vi "OutputSwerveAzimuth.vi"() -> ()   [LabVIEW 2020]
doc: "This VI runs feedback and feedforward controllers, manages safety interlocks, and sends commands to the swerve azimuth motors."
uses:
  <vilib>/Rock Robotics/WPI/ThirdParty/Phoenix-LabVIEW/Motor Controller/Controls/CTRE_Phoenix_MotorControl_ControlMode.ctl
  <vilib>/Rock Robotics/WPI/ThirdParty/Phoenix-LabVIEW/Motor Controller/Controls/CTRE_Phoenix_MotorControl_NeutralMode.ctl
  6e813111-160f-47d9-be7e-04f12fb0a952.vi
  refnumbers.vi
  GRNF_CTREMotor.vi
  sensordata.vi
  driverdata.vi
  robotoutputs.vi
  robotconstants.vi
  TAI_Motor.vi
  <vilib>/Rock Robotics/WPI/ThirdParty/Phoenix-LabVIEW/Motor Controller/Get/CTRE_Phoenix_MotorController_GetSelectedSensorData.vi
panel:
  out "Azimuth Error (deg)":dbl
  out "Azimuth Velocity":cluster{dbl}(graph)
  out "Azimuth Position":cluster{dbl, "Interlock Output":dbl}(graph)
  in  "PID Parameters":T1={"Kp"=0.3, "Ki"=0.0, "Kd"=0.0, "Kf (don't use)"=0.0, "I-Zone"=10.0} {"Kd" min=0.0; "Ki" min=0.0; "Kp" min=0.0}
  in  "S-Curve Strength":i32=4
  in  "Acceleration (deg/s^2)":dbl=10000.0
  in  "Cruise Velocity (deg/s)":dbl=1000.0
  in  "Manual Azimuth Goal (deg) [-180,180]":dbl
  in  "Manually Override Azimuth Goal":bool
  in  "Best Angle Hysteresis (deg)":dbl=20.0 format="%#_13g"
  in  "Plotting":T2(ring)
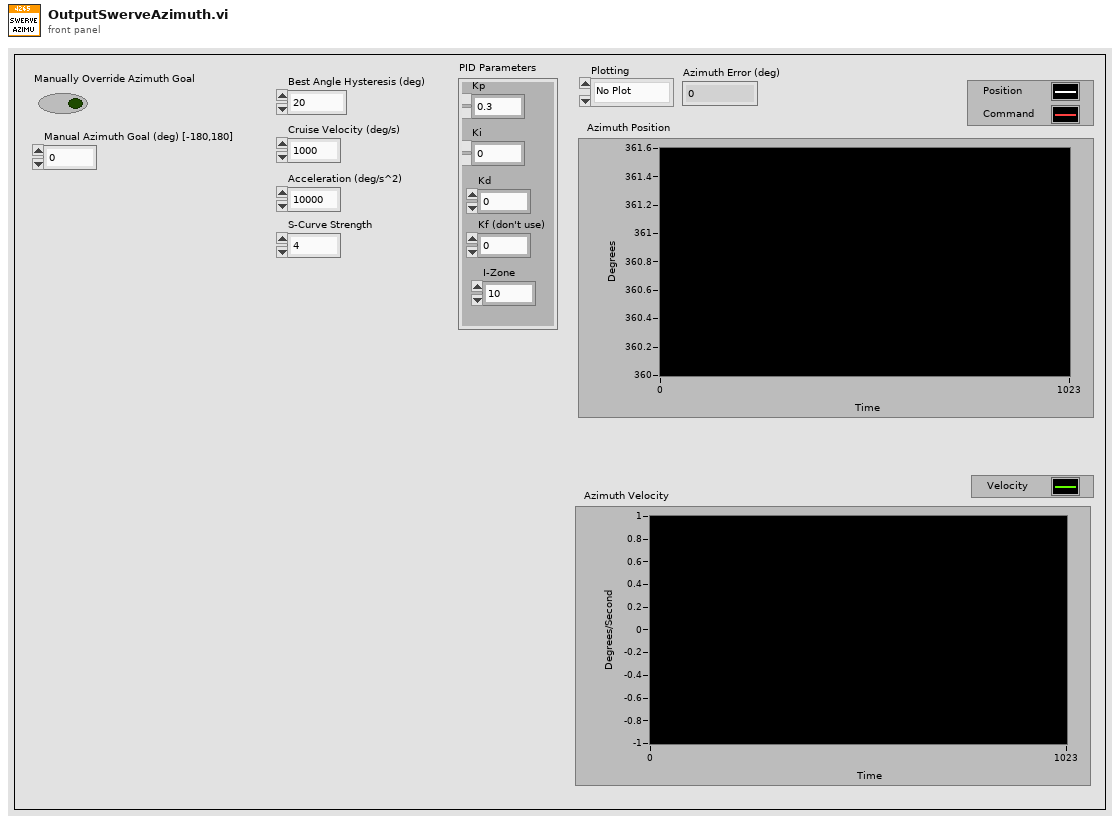
[diagram p1: front panel]
types:
  T1 = cluster{"Kp":dbl, "Ki":dbl, "Kd":dbl, "Kf (don't use)":dbl, "I-Zone":dbl}
  T2 = enum16{"No Plot", "Module 0", "Module 1", "Module 2", "Module 3"}
  T3 = cluster{"Cruise Velocity (deg/s)":i32, "Acceleration (deg/s^2)":i32, "S-Curve Strength":i32}
  T4 = cluster{"Cruise Velocity (deg/s)":bool, "Acceleration (deg/s^2)":bool, "S-Curve Strength":bool}
  T5 = cluster{"Kp":bool, "Ki":bool, "Kd":bool, "Kf (don't use)":bool, "I-Zone":bool}
  T6 = typedef "WPI_MotorControlDeviceRef.ctl" = cluster{"DeviceStatus":errorcluster, "Type":T7, "PWM":cluster{"PWM Channel":T8, "DeadBand":T9}, "CAN":cluster{"Device Number":u8, "SetOutput VI Ref":variant, "GetOutput VI Ref":variant, "Enable VI Ref":variant, "Disable VI Ref":variant, "Data":variant}, "Invert":bool, "DIO PWM":cluster{"PWM \"Enable\" Channel":T8, "DIOChannel":T10, "PWM Rate":dbl}}
  T7 = typedef "WPI_MotorControlType.ctl" = enum16{"PWM", "CAN", "DIO PWM"}
  T8 = typedef "FPGA_DIOPWMChannel.ctl" = enum8{"PWM 0", "PWM 1", "PWM 2", "PWM 3", "PWM 4", "PWM 5", "PWM 6", "PWM 7", "PWM 8", "PWM 9", "PWM MXP 0", "PWM MXP 1", "PWM MXP 2", "PWM MXP 3", "PWM MXP 4", "PWM MXP 5", "PWM MXP 6", "PWM MXP 7", "PWM MXP 8", "PWM MXP 9", "Invalid"}
  T9 = typedef "WPI_PWMDeadband.ctl" = cluster{"Name":string, "maxPositivePwm":i32, "minPositivePwm":i32, "centerPwm":i32, "maxNegativePwm":i32, "minNegativePwm":i32, "angularRange":u16}
  T10 = typedef "FPGA_DIOChannel.ctl" = enum8{"DIO 0", "DIO 1", "DIO 2", "DIO 3", "DIO 4", "DIO 5", "DIO 6", "DIO 7", "DIO 8", "DIO 9", "DIO MXP 0", "DIO MXP 1", "DIO MXP 2", "DIO MXP 3", "DIO MXP 4", "DIO MXP 5", "DIO MXP 6", "DIO MXP 7", "DIO MXP 8", "DIO MXP 9", "DIO MXP 10", "DIO MXP 11", "DIO MXP 12", "DIO MXP 13", "DIO MXP 14", "DIO MXP 15", "SPI Port CS1", "SPI Port CS2", "SPI Port CS3", "SPI Port MISO", "SPI Port MOSI", "Invalid"}
  T11 = typedef "CTRE_Phoenix_MotorControl_NeutralMode.ctl" = enum8{"EEPROMSetting", "Override to Coast", "Override to Brake"}
  T12 = typedef "CTRE_Phoenix_MotorControl_ControlMode.ctl" = u16
  T13 = enum16{"No Changed Output", "New Normal Output", "New Testing Output"}
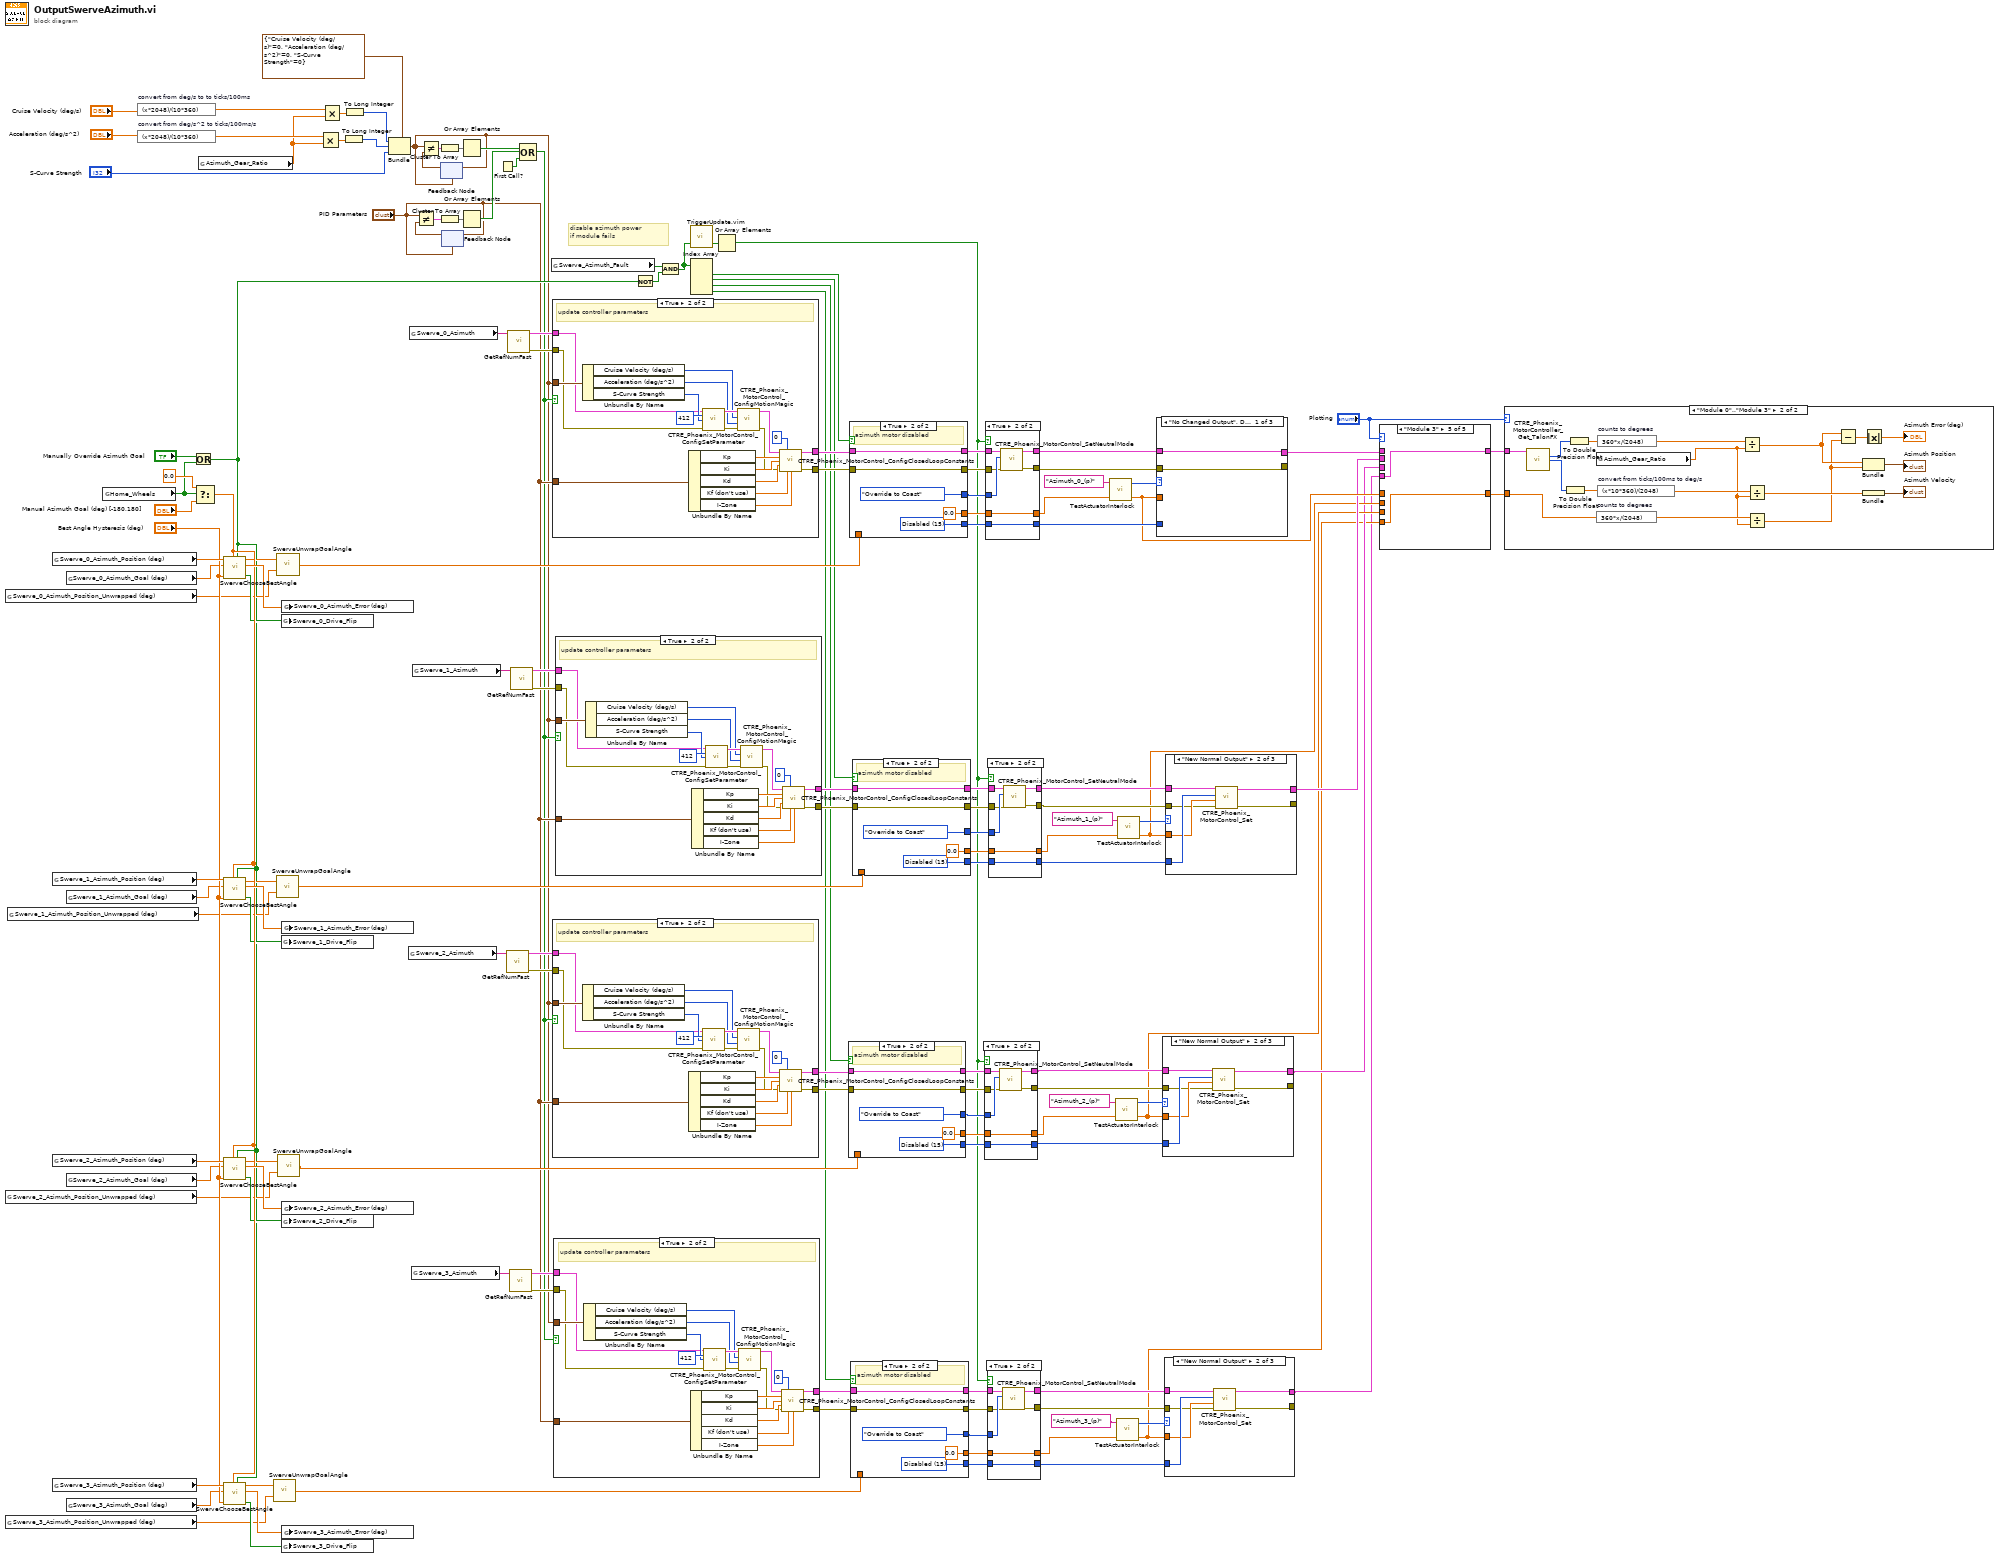
[diagram p0: block diagram]
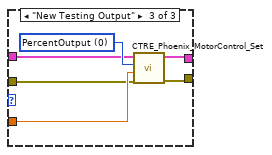
[diagram p3: hidden frame]
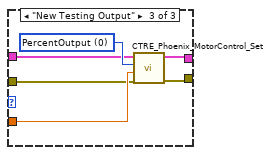
[diagram p5: hidden frame]
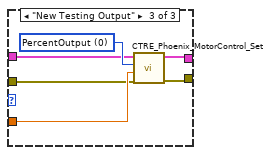
[diagram p7: hidden frame]
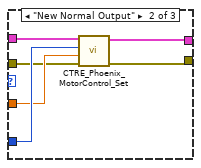
[diagram p8: hidden frame]
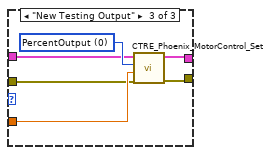
[diagram p9: hidden frame]
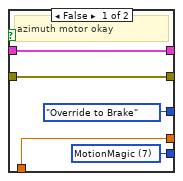
[diagram p12: hidden frame]
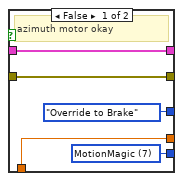
[diagram p15: hidden frame]
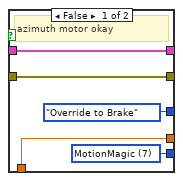
[diagram p18: hidden frame]
diagram:
  # "disable azimuth power\nif module fails"
  n1 = global read "sensordata.vi" "Swerve_0_Azimuth_Position_Unwrapped (deg)"() -> (w93:dbl)
  n2 = global read "sensordata.vi" "Swerve_2_Azimuth_Position_Unwrapped (deg)"() -> (w90:dbl)
  n3 = global read "sensordata.vi" "Swerve_3_Azimuth_Position_Unwrapped (deg)"() -> (w88:dbl)
  n4 = global read "sensordata.vi" "Swerve_1_Azimuth_Position_Unwrapped (deg)"() -> (w92:dbl)
  n5 = global read "sensordata.vi" "Swerve_0_Azimuth_Position (deg)"() -> (w131:dbl)
  n6 = global read "sensordata.vi" "Swerve_1_Azimuth_Position (deg)"() -> (w130:dbl)
  n7 = global read "sensordata.vi" "Swerve_2_Azimuth_Position (deg)"() -> (w129:dbl)
  n8 = global read "sensordata.vi" "Swerve_3_Azimuth_Position (deg)"() -> (w128:dbl)
  n9 = global read "robotoutputs.vi" "Swerve_0_Azimuth_Goal (deg)"() -> (w125:dbl)
  n10 = global read "robotoutputs.vi" "Swerve_1_Azimuth_Goal (deg)"() -> (w124:dbl)
  n11 = global read "robotoutputs.vi" "Swerve_2_Azimuth_Goal (deg)"() -> (w123:dbl)
  n12 = global read "robotoutputs.vi" "Swerve_3_Azimuth_Goal (deg)"() -> (w122:dbl)
  n13 = global read "driverdata.vi" "Home_Wheels"() -> (w136:bool)
  n14 = expression code="(x*2048)/(10*360)" "convert from deg/s to to ticks/100ms"("Cruise Velocity (deg/s)") -> (w7:dbl)
  n15 = expression code="(x*2048)/(10*360)" "convert from deg/s^2 to ticks/100ms/s"("Acceleration (deg/s^2)") -> (w8:dbl)
  n16 = Or(x="Manually Override Azimuth Goal", y=w136) -> (x .or. y?=w83:bool)
  n17 = Select(t=0.0 ("f"), s=w136, f="Manual Azimuth Goal (deg) [-180,180]") -> (s? t:f=w127:dbl)
  n18 = global read "robotconstants.vi" "Azimuth_Gear_Ratio"() -> (w6:dbl)
  n19 = call "SwerveChooseBestAngle.vi"("Goal Override"=w83, "Goal Override Angle (deg) [-180,+180]"=w127, "Hysteresis (deg)"="Best Angle Hysteresis (deg)", "Goal Angle (deg) [-180,+180]"=w125, "Current Angle (deg) [-180,+180]"=w131) -> ("Flip Drive Motor Direction"=w121:bool, "Flipped Angular Distance (deg)"=w135:dbl, "Flipped Goal Angle (deg) [-180, +180]"=w117:dbl)  [unwired: 4 in]
  n20 = call "SwerveChooseBestAngle.vi"("Goal Override"=w83, "Goal Override Angle (deg) [-180,+180]"=w127, "Hysteresis (deg)"="Best Angle Hysteresis (deg)", "Goal Angle (deg) [-180,+180]"=w124, "Current Angle (deg) [-180,+180]"=w130) -> ("Flip Drive Motor Direction"=w120:bool, "Flipped Angular Distance (deg)"=w134:dbl, "Flipped Goal Angle (deg) [-180, +180]"=w91:dbl)  [unwired: 4 in]
  n21 = call "SwerveChooseBestAngle.vi"("Goal Override"=w83, "Goal Override Angle (deg) [-180,+180]"=w127, "Hysteresis (deg)"="Best Angle Hysteresis (deg)", "Goal Angle (deg) [-180,+180]"=w123, "Current Angle (deg) [-180,+180]"=w129) -> ("Flip Drive Motor Direction"=w119:bool, "Flipped Angular Distance (deg)"=w133:dbl, "Flipped Goal Angle (deg) [-180, +180]"=w89:dbl)  [unwired: 4 in]
  n22 = call "SwerveChooseBestAngle.vi"("Goal Override"=w83, "Goal Override Angle (deg) [-180,+180]"=w127, "Hysteresis (deg)"="Best Angle Hysteresis (deg)", "Goal Angle (deg) [-180,+180]"=w122, "Current Angle (deg) [-180,+180]"=w128) -> ("Flip Drive Motor Direction"=w118:bool, "Flipped Angular Distance (deg)"=w132:dbl, "Flipped Goal Angle (deg) [-180, +180]"=w87:dbl)  [unwired: 4 in]
  n23 = call "SwerveUnwrapGoalAngle.vi"("Current Unwrapped Angle (deg) [-Inf,+Inf]"=w88, "Flipped Goal Angle (deg) [-180, +180]"=w87) -> ("Absolute Azimuth Position (tics) [-Inf,+Inf]"=w48:dbl)
  n24 = call "SwerveUnwrapGoalAngle.vi"("Current Unwrapped Angle (deg) [-Inf,+Inf]"=w92, "Flipped Goal Angle (deg) [-180, +180]"=w91) -> ("Absolute Azimuth Position (tics) [-Inf,+Inf]"=w71:dbl)
  n25 = call "SwerveUnwrapGoalAngle.vi"("Current Unwrapped Angle (deg) [-Inf,+Inf]"=w93, "Flipped Goal Angle (deg) [-180, +180]"=w117) -> ("Absolute Azimuth Position (tics) [-Inf,+Inf]"=w96:dbl)
  n26 = call "SwerveUnwrapGoalAngle.vi"("Current Unwrapped Angle (deg) [-Inf,+Inf]"=w90, "Flipped Goal Angle (deg) [-180, +180]"=w89) -> ("Absolute Azimuth Position (tics) [-Inf,+Inf]"=w60:dbl)
  n27 = global write "robotoutputs.vi" "Swerve_0_Drive_Flip"(w121) -> ()
  n28 = global write "robotoutputs.vi" "Swerve_1_Drive_Flip"(w120) -> ()
  n29 = global write "robotoutputs.vi" "Swerve_2_Drive_Flip"(w119) -> ()
  n30 = global write "robotoutputs.vi" "Swerve_3_Drive_Flip"(w118) -> ()
  n31 = global write "robotoutputs.vi" "Swerve_0_Azimuth_Error (deg)"(w135) -> ()
  n32 = global write "robotoutputs.vi" "Swerve_1_Azimuth_Error (deg)"(w134) -> ()
  n33 = global write "robotoutputs.vi" "Swerve_2_Azimuth_Error (deg)"(w133) -> ()
  n34 = global write "robotoutputs.vi" "Swerve_3_Azimuth_Error (deg)"(w132) -> ()
  n35 = Multiply(x=w8, y=w6) -> (x*y=w9:dbl)
  n36 = Multiply(x=w7, y=w6) -> (x*y=w10:dbl)
  n37 = To Long Integer(number=w9) -> (32bit integer=w2:i32)
  n38 = To Long Integer(number=w10) -> (32bit integer=w1:i32)
  n39 = Bundle(cluster=T3 {"Cruise Velocity (deg/s)"=0, "Acceleration (deg/s^2)"=0, "S-Curve Strength"=0}, "Cruise Velocity (deg/s)"=w1, "Acceleration (deg/s^2)"=w2, "S-Curve Strength"="S-Curve Strength") -> (w45:T3)
  n40 = global read "refnumbers.vi" "Swerve_2_Azimuth"() -> (w70:string)
  n41 = global read "refnumbers.vi" "Swerve_0_Azimuth"() -> (w141:string)
  n42 = global read "refnumbers.vi" "Swerve_3_Azimuth"() -> (w58:string)
  n43 = global read "refnumbers.vi" "Swerve_1_Azimuth"() -> (w82:string)
  n44 = feedback #1(w45) -> (w110:T3)
  n45 = Not Equal?(x=w45, y=w110) -> (x != y?=w112:T4)
  n46 = Cluster To Array(cluster=w112) -> (array=w111:bool[])
  n47 = feedback-in #1(w45) -> ()
  n48 = feedback #2("PID Parameters") -> (w114:T1)
  n49 = Not Equal?(x="PID Parameters", y=w114) -> (x != y?=w116:T5)
  n50 = Cluster To Array(cluster=w116) -> (array=w115:bool[])
  n51 = feedback-in #2("PID Parameters") -> ()
  n52 = Or Array Elements(Boolean array=w111) -> (logical OR=w109:bool)
  n53 = Or Array Elements(Boolean array=w115) -> (logical OR=w108:bool)
  n54 = First Call?() -> (First Call?: T/F=w107:bool)
  n55 = call-poly "GetRefNumFast.vi"("RefNum Name"=w70) -> ("Error"=w68:errorcluster, "Device Reference"=w69:T6)  [unwired: 5 in]
  n56 = call-poly "GetRefNumFast.vi"("RefNum Name"=w141) -> ("Error"=w105:errorcluster, "Device Reference"=w106:T6)  [unwired: 5 in]
  n57 = call-poly "GetRefNumFast.vi"("RefNum Name"=w58) -> ("Error"=w56:errorcluster, "Device Reference"=w57:T6)  [unwired: 5 in]
  n58 = call-poly "GetRefNumFast.vi"("RefNum Name"=w82) -> ("Error"=w80:errorcluster, "Device Reference"=w81:T6)  [unwired: 5 in]
  n59 = Compound Arithmetic op=OR(w109, w108, w107) -> (w46:bool)
  n60 = global read "sensordata.vi" "Swerve_Azimuth_Fault"() -> (w86:bool[])
  n61 = case shown="True" w46 {
    tunnel: w45 -> [_ w161]
    tunnel: "PID Parameters" -> [_ w153]
    tunnel: [w144 w148] -> w104
    tunnel: [w143 w147] -> w103
    tunnel: w106 -> [w144 w146]
    tunnel: w105 -> [w143 w145]
    frame False {
      # "holde controller parameters"
    }
    frame True {
      # "update controller parameters"
      n62 = Unbundle By Name(w161) -> ("Cruise Velocity (deg/s)"=w158:i32, "Acceleration (deg/s^2)"=w159:i32, "S-Curve Strength"=w160:i32)
      n63 = Unbundle By Name(w153) -> ("Kp"=w157:dbl, "Ki"=w156:dbl, "Kd"=w155:dbl, "Kf (don't use)"=w152:dbl, "I-Zone"=w151:dbl)
      n64 = call <vilib>:"CTRE_Phoenix_MotorControl_ConfigSetParameter.vi"("PhoenixMotorControlDevRef"=w146, "Parameter"=412 ("New Sensor Position"), "value"=w160, "error in (no error)"=w145) -> ("PhoenixMotorControlDevRef"=w163:T6, "error out"=w162:errorcluster)  [unwired: 10 in]
      n65 = call <vilib>:"CTRE_Phoenix_MotorControl_ConfigMotionMagic.vi"("error in (no error)"=w162, "Acceleration"=w159, "Cruise Velocity"=w158, "PhoenixMotorControlDevRef"=w163) -> ("error out"=w149:errorcluster, "PhoenixMotorControlDevRef"=w150:T6)  [unwired: 6 in]
      n66 = call <vilib>:"CTRE_Phoenix_MotorControl_ConfigClosedLoopConstants.vi"("PhoenixMotorControlDevRef"=w150, "slotIdx"=0, "P"=w157, "I"=w156, "D"=w155, "error in (no error)"=w149, "F"=w152, "I Zone"=w151) -> ("PhoenixMotorControlDevRef"=w148:T6, "error out"=w147:errorcluster)  [unwired: 6 in]
    }
  }
  n67 = case shown="True" w46 {
    tunnel: w45 -> [_ w183]
    tunnel: "PID Parameters" -> [_ w175]
    tunnel: [w166 w170] -> w67
    tunnel: [w165 w169] -> w66
    tunnel: w69 -> [w166 w168]
    tunnel: w68 -> [w165 w167]
    frame False {
      # "holde controller parameters"
    }
    frame True {
      # "update controller parameters"
      n68 = Unbundle By Name(w183) -> ("Cruise Velocity (deg/s)"=w180:i32, "Acceleration (deg/s^2)"=w181:i32, "S-Curve Strength"=w182:i32)
      n69 = Unbundle By Name(w175) -> ("Kp"=w179:dbl, "Ki"=w178:dbl, "Kd"=w177:dbl, "Kf (don't use)"=w174:dbl, "I-Zone"=w173:dbl)
      n70 = call <vilib>:"CTRE_Phoenix_MotorControl_ConfigSetParameter.vi"("PhoenixMotorControlDevRef"=w168, "Parameter"=412 ("New Sensor Position"), "value"=w182, "error in (no error)"=w167) -> ("PhoenixMotorControlDevRef"=w185:T6, "error out"=w184:errorcluster)  [unwired: 10 in]
      n71 = call <vilib>:"CTRE_Phoenix_MotorControl_ConfigMotionMagic.vi"("error in (no error)"=w184, "Acceleration"=w181, "Cruise Velocity"=w180, "PhoenixMotorControlDevRef"=w185) -> ("error out"=w171:errorcluster, "PhoenixMotorControlDevRef"=w172:T6)  [unwired: 6 in]
      n72 = call <vilib>:"CTRE_Phoenix_MotorControl_ConfigClosedLoopConstants.vi"("PhoenixMotorControlDevRef"=w172, "slotIdx"=0, "P"=w179, "I"=w178, "D"=w177, "error in (no error)"=w171, "F"=w174, "I Zone"=w173) -> ("PhoenixMotorControlDevRef"=w170:T6, "error out"=w169:errorcluster)  [unwired: 6 in]
    }
  }
  n73 = case shown="True" w46 {
    tunnel: w45 -> [_ w205]
    tunnel: "PID Parameters" -> [_ w197]
    tunnel: [w188 w192] -> w55
    tunnel: [w187 w191] -> w54
    tunnel: w57 -> [w188 w190]
    tunnel: w56 -> [w187 w189]
    frame False {
      # "holde controller parameters"
    }
    frame True {
      # "update controller parameters"
      n74 = Unbundle By Name(w205) -> ("Cruise Velocity (deg/s)"=w202:i32, "Acceleration (deg/s^2)"=w203:i32, "S-Curve Strength"=w204:i32)
      n75 = Unbundle By Name(w197) -> ("Kp"=w201:dbl, "Ki"=w200:dbl, "Kd"=w199:dbl, "Kf (don't use)"=w196:dbl, "I-Zone"=w195:dbl)
      n76 = call <vilib>:"CTRE_Phoenix_MotorControl_ConfigSetParameter.vi"("PhoenixMotorControlDevRef"=w190, "Parameter"=412 ("New Sensor Position"), "value"=w204, "error in (no error)"=w189) -> ("PhoenixMotorControlDevRef"=w207:T6, "error out"=w206:errorcluster)  [unwired: 10 in]
      n77 = call <vilib>:"CTRE_Phoenix_MotorControl_ConfigMotionMagic.vi"("error in (no error)"=w206, "Acceleration"=w203, "Cruise Velocity"=w202, "PhoenixMotorControlDevRef"=w207) -> ("error out"=w193:errorcluster, "PhoenixMotorControlDevRef"=w194:T6)  [unwired: 6 in]
      n78 = call <vilib>:"CTRE_Phoenix_MotorControl_ConfigClosedLoopConstants.vi"("PhoenixMotorControlDevRef"=w194, "slotIdx"=0, "P"=w201, "I"=w200, "D"=w199, "error in (no error)"=w193, "F"=w196, "I Zone"=w195) -> ("PhoenixMotorControlDevRef"=w192:T6, "error out"=w191:errorcluster)  [unwired: 6 in]
    }
  }
  n79 = case shown="True" w46 {
    tunnel: w45 -> [_ w227]
    tunnel: "PID Parameters" -> [_ w219]
    tunnel: [w210 w214] -> w79
    tunnel: [w209 w213] -> w78
    tunnel: w81 -> [w210 w212]
    tunnel: w80 -> [w209 w211]
    frame False {
      # "holde controller parameters"
    }
    frame True {
      # "update controller parameters"
      n80 = Unbundle By Name(w227) -> ("Cruise Velocity (deg/s)"=w224:i32, "Acceleration (deg/s^2)"=w225:i32, "S-Curve Strength"=w226:i32)
      n81 = Unbundle By Name(w219) -> ("Kp"=w223:dbl, "Ki"=w222:dbl, "Kd"=w221:dbl, "Kf (don't use)"=w218:dbl, "I-Zone"=w217:dbl)
      n82 = call <vilib>:"CTRE_Phoenix_MotorControl_ConfigSetParameter.vi"("PhoenixMotorControlDevRef"=w212, "Parameter"=412 ("New Sensor Position"), "value"=w226, "error in (no error)"=w211) -> ("PhoenixMotorControlDevRef"=w229:T6, "error out"=w228:errorcluster)  [unwired: 10 in]
      n83 = call <vilib>:"CTRE_Phoenix_MotorControl_ConfigMotionMagic.vi"("error in (no error)"=w228, "Acceleration"=w225, "Cruise Velocity"=w224, "PhoenixMotorControlDevRef"=w229) -> ("error out"=w215:errorcluster, "PhoenixMotorControlDevRef"=w216:T6)  [unwired: 6 in]
      n84 = call <vilib>:"CTRE_Phoenix_MotorControl_ConfigClosedLoopConstants.vi"("PhoenixMotorControlDevRef"=w216, "slotIdx"=0, "P"=w223, "I"=w222, "D"=w221, "error in (no error)"=w215, "F"=w218, "I Zone"=w217) -> ("PhoenixMotorControlDevRef"=w214:T6, "error out"=w213:errorcluster)  [unwired: 6 in]
    }
  }
  n85 = Not(x=w83) -> (.not. x?=w84:bool)
  n86 = And(x=w86, y=w84) -> (x .and. y?=w85:bool[])
  n87 = call "TriggerUpdate.vim"("Trigger"=w85) -> ("Update"=w99:bool[])  [unwired: 2 in]
  n88 = Index Array(array=w85) -> (element #1=w142:bool, element #2=w72:bool, element #3=w59:bool, element #4=w44:bool)  [unwired: 4 in]
  n89 = Or Array Elements(Boolean array=w99) -> (logical OR=w43:bool)
  n90 = case shown="True" w59 {
    tunnel: [w235 w240] -> w64
    tunnel: w67 -> [w235 w240]
    tunnel: [w231 0.0 ("Command")] -> w62
    tunnel: [w234 w238] -> w61
    tunnel: [CTRE_Phoenix_MotorControl_NeutralMode."Override to Brake" ("Motor Control Neutral Mode") CTRE_Phoenix_MotorControl_NeutralMode."Override to Coast" ("Motor Control Neutral Mode")] -> w65
    tunnel: w66 -> [w232 w236]
    tunnel: [w232 w236] -> w63
    tunnel: w60 -> [w231 _]
    frame False {
      w234 = T12 7 items=["PercentOutput"=0, "Position"=1, "Velocity"=2, "Current"=3, "Follower"=5, "MotionProfile"=6, "MotionMagic"=7, "MotionProfileArc"=10, "Disabled"=15] ("Control Mode")
      # "azimuth motor okay"
    }
    frame True {
      w238 = T12 15 items=["PercentOutput"=0, "Position"=1, "Velocity"=2, "Current"=3, "Follower"=5, "MotionProfile"=6, "MotionMagic"=7, "MotionProfileArc"=10, "Disabled"=15] ("Control Mode")
      # "azimuth motor disabled"
    }
  }
  n91 = case shown="True" w142 {
    tunnel: [w245 w250] -> w101
    tunnel: w104 -> [w245 w250]
    tunnel: [w241 0.0 ("Command")] -> w98
    tunnel: [w244 w248] -> w97
    tunnel: [CTRE_Phoenix_MotorControl_NeutralMode."Override to Brake" ("Motor Control Neutral Mode") CTRE_Phoenix_MotorControl_NeutralMode."Override to Coast" ("Motor Control Neutral Mode")] -> w102
    tunnel: w103 -> [w242 w246]
    tunnel: [w242 w246] -> w100
    tunnel: w96 -> [w241 _]
    frame False {
      w244 = T12 7 items=["PercentOutput"=0, "Position"=1, "Velocity"=2, "Current"=3, "Follower"=5, "MotionProfile"=6, "MotionMagic"=7, "MotionProfileArc"=10, "Disabled"=15] ("Control Mode")
      # "azimuth motor okay"
    }
    frame True {
      w248 = T12 15 items=["PercentOutput"=0, "Position"=1, "Velocity"=2, "Current"=3, "Follower"=5, "MotionProfile"=6, "MotionMagic"=7, "MotionProfileArc"=10, "Disabled"=15] ("Control Mode")
      # "azimuth motor disabled"
    }
  }
  n92 = case shown="True" w44 {
    tunnel: [w255 w260] -> w52
    tunnel: w55 -> [w255 w260]
    tunnel: [w251 0.0 ("Command")] -> w50
    tunnel: [w254 w258] -> w49
    tunnel: [CTRE_Phoenix_MotorControl_NeutralMode."Override to Brake" ("Motor Control Neutral Mode") CTRE_Phoenix_MotorControl_NeutralMode."Override to Coast" ("Motor Control Neutral Mode")] -> w53
    tunnel: w54 -> [w252 w256]
    tunnel: [w252 w256] -> w51
    tunnel: w48 -> [w251 _]
    frame False {
      w254 = T12 7 items=["PercentOutput"=0, "Position"=1, "Velocity"=2, "Current"=3, "Follower"=5, "MotionProfile"=6, "MotionMagic"=7, "MotionProfileArc"=10, "Disabled"=15] ("Control Mode")
      # "azimuth motor okay"
    }
    frame True {
      w258 = T12 15 items=["PercentOutput"=0, "Position"=1, "Velocity"=2, "Current"=3, "Follower"=5, "MotionProfile"=6, "MotionMagic"=7, "MotionProfileArc"=10, "Disabled"=15] ("Control Mode")
      # "azimuth motor disabled"
    }
  }
  n93 = case shown="True" w72 {
    tunnel: [w265 w270] -> w76
    tunnel: w79 -> [w265 w270]
    tunnel: [w261 0.0 ("Command")] -> w74
    tunnel: [w264 w268] -> w73
    tunnel: [CTRE_Phoenix_MotorControl_NeutralMode."Override to Brake" ("Motor Control Neutral Mode") CTRE_Phoenix_MotorControl_NeutralMode."Override to Coast" ("Motor Control Neutral Mode")] -> w77
    tunnel: w78 -> [w262 w266]
    tunnel: [w262 w266] -> w75
    tunnel: w71 -> [w261 _]
    frame False {
      w264 = T12 7 items=["PercentOutput"=0, "Position"=1, "Velocity"=2, "Current"=3, "Follower"=5, "MotionProfile"=6, "MotionMagic"=7, "MotionProfileArc"=10, "Disabled"=15] ("Control Mode")
      # "azimuth motor okay"
    }
    frame True {
      w268 = T12 15 items=["PercentOutput"=0, "Position"=1, "Velocity"=2, "Current"=3, "Follower"=5, "MotionProfile"=6, "MotionMagic"=7, "MotionProfileArc"=10, "Disabled"=15] ("Control Mode")
      # "azimuth motor disabled"
    }
  }
  n94 = case shown="True" w43 {
    tunnel: w65 -> [_ w281]
    tunnel: w64 -> [w274 w280]
    tunnel: w63 -> [w273 w279]
    tunnel: [w274 w278] -> w24
    tunnel: [w273 w277] -> w23
    tunnel: w62 -> [w272 w276]
    tunnel: [w272 w276] -> w22
    tunnel: w61 -> [w271 w275]
    tunnel: [w271 w275] -> w21
    frame False {
    }
    frame True {
      n95 = call <vilib>:"CTRE_Phoenix_MotorControl_SetNeutralMode.vi"("error in (no error)"=w279, "Motor Control Neutral Mode"=w281, "PhoenixMotorControlDevRef"=w280) -> ("error out"=w277:errorcluster, "PhoenixMotorControlDevRef"=w278:T6)  [unwired: 7 in]
    }
  }
  n96 = case shown="True" w43 {
    tunnel: w102 -> [_ w292]
    tunnel: w101 -> [w285 w291]
    tunnel: w100 -> [w284 w290]
    tunnel: [w285 w289] -> w40
    tunnel: [w284 w288] -> w39
    tunnel: w98 -> [w283 w287]
    tunnel: [w283 w287] -> w37
    tunnel: w97 -> [w282 w286]
    tunnel: [w282 w286] -> w38
    frame False {
    }
    frame True {
      n97 = call <vilib>:"CTRE_Phoenix_MotorControl_SetNeutralMode.vi"("error in (no error)"=w290, "Motor Control Neutral Mode"=w292, "PhoenixMotorControlDevRef"=w291) -> ("error out"=w288:errorcluster, "PhoenixMotorControlDevRef"=w289:T6)  [unwired: 7 in]
    }
  }
  n98 = case shown="True" w43 {
    tunnel: w53 -> [_ w303]
    tunnel: w52 -> [w296 w302]
    tunnel: w51 -> [w295 w301]
    tunnel: [w296 w300] -> w16
    tunnel: [w295 w299] -> w15
    tunnel: w50 -> [w294 w298]
    tunnel: [w294 w298] -> w14
    tunnel: w49 -> [w293 w297]
    tunnel: [w293 w297] -> w13
    frame False {
    }
    frame True {
      n99 = call <vilib>:"CTRE_Phoenix_MotorControl_SetNeutralMode.vi"("error in (no error)"=w301, "Motor Control Neutral Mode"=w303, "PhoenixMotorControlDevRef"=w302) -> ("error out"=w299:errorcluster, "PhoenixMotorControlDevRef"=w300:T6)  [unwired: 7 in]
    }
  }
  n100 = case shown="True" w43 {
    tunnel: w77 -> [_ w314]
    tunnel: w76 -> [w307 w313]
    tunnel: w75 -> [w306 w312]
    tunnel: [w307 w311] -> w29
    tunnel: [w306 w310] -> w30
    tunnel: w74 -> [w305 w309]
    tunnel: [w305 w309] -> w31
    tunnel: w73 -> [w304 w308]
    tunnel: [w304 w308] -> w32
    frame False {
    }
    frame True {
      n101 = call <vilib>:"CTRE_Phoenix_MotorControl_SetNeutralMode.vi"("error in (no error)"=w312, "Motor Control Neutral Mode"=w314, "PhoenixMotorControlDevRef"=w313) -> ("error out"=w310:errorcluster, "PhoenixMotorControlDevRef"=w311:T6)  [unwired: 7 in]
    }
  }
  n102 = call-poly "TestActuatorInterlock.vi"("Normal Output"=w37, "Actuator Name"="Azimuth_0_(p)" ("Actuator_Name")) -> ("Interlocked Output"=w36:dbl, "Output Mode"=w42:T13)  [unwired: 2 in]
  n103 = call-poly "TestActuatorInterlock.vi"("Normal Output"=w22, "Actuator Name"="Azimuth_2_(p)" ("Actuator_Name")) -> ("Interlocked Output"=w20:dbl, "Output Mode"=w26:T13)  [unwired: 2 in]
  n104 = call-poly "TestActuatorInterlock.vi"("Normal Output"=w14, "Actuator Name"="Azimuth_3_(p)" ("Actuator_Name")) -> ("Interlocked Output"=w12:dbl, "Output Mode"=w18:T13)  [unwired: 2 in]
  n105 = call-poly "TestActuatorInterlock.vi"("Normal Output"=w31, "Actuator Name"="Azimuth_1_(p)" ("Actuator_Name")) -> ("Interlocked Output"=w27:dbl, "Output Mode"=w34:T13)  [unwired: 2 in]
  n106 = case shown="\"No Changed Output\", Default" w42 {
    tunnel: w38 -> [_ w322 _]
    tunnel: w40 -> [w316 w320 w327]
    tunnel: w36 -> [_ w321 w326]
    tunnel: w39 -> [w315 w317 w325]
    tunnel: [w316 w319 w324] -> w35
    tunnel: [w315 w318 w323] -> _
    frame "No Changed Output", Default {
    }
    frame "New Normal Output" {
      n107 = call <vilib>:"CTRE_Phoenix_MotorControl_Set.vi"("error in (no error)"=w317, "Output"=w321, "Control Mode"=w322, "PhoenixMotorControlDevRef"=w320) -> ("error out"=w318:errorcluster, "PhoenixMotorControlDevRef"=w319:T6)  [unwired: 6 in]
    }
    frame "New Testing Output" {
      w328 = T12 0 items=["PercentOutput"=0, "Position"=1, "Velocity"=2, "Current"=3, "Follower"=5, "MotionProfile"=6, "MotionMagic"=7, "MotionProfileArc"=10, "Disabled"=15] ("Control Mode")
      n108 = call <vilib>:"CTRE_Phoenix_MotorControl_Set.vi"("error in (no error)"=w325, "Output"=w326, "Control Mode"=w328, "PhoenixMotorControlDevRef"=w327) -> ("error out"=w323:errorcluster, "PhoenixMotorControlDevRef"=w324:T6)  [unwired: 6 in]
    }
  }
  n109 = case shown="\"New Normal Output\"" w26 {
    tunnel: w21 -> [_ w336 _]
    tunnel: w24 -> [w330 w334 w341]
    tunnel: w20 -> [_ w335 w340]
    tunnel: w23 -> [w329 w331 w339]
    tunnel: [w330 w333 w338] -> w19
    tunnel: [w329 w332 w337] -> _
    frame "No Changed Output", Default {
    }
    frame "New Normal Output" {
      n110 = call <vilib>:"CTRE_Phoenix_MotorControl_Set.vi"("error in (no error)"=w331, "Output"=w335, "Control Mode"=w336, "PhoenixMotorControlDevRef"=w334) -> ("error out"=w332:errorcluster, "PhoenixMotorControlDevRef"=w333:T6)  [unwired: 6 in]
    }
    frame "New Testing Output" {
      w342 = T12 0 items=["PercentOutput"=0, "Position"=1, "Velocity"=2, "Current"=3, "Follower"=5, "MotionProfile"=6, "MotionMagic"=7, "MotionProfileArc"=10, "Disabled"=15] ("Control Mode")
      n111 = call <vilib>:"CTRE_Phoenix_MotorControl_Set.vi"("error in (no error)"=w339, "Output"=w340, "Control Mode"=w342, "PhoenixMotorControlDevRef"=w341) -> ("error out"=w337:errorcluster, "PhoenixMotorControlDevRef"=w338:T6)  [unwired: 6 in]
    }
  }
  n112 = case shown="\"New Normal Output\"" w18 {
    tunnel: w13 -> [_ w350 _]
    tunnel: w16 -> [w344 w348 w355]
    tunnel: w12 -> [_ w349 w354]
    tunnel: w15 -> [w343 w345 w353]
    tunnel: [w344 w347 w352] -> w11
    tunnel: [w343 w346 w351] -> _
    frame "No Changed Output", Default {
    }
    frame "New Normal Output" {
      n113 = call <vilib>:"CTRE_Phoenix_MotorControl_Set.vi"("error in (no error)"=w345, "Output"=w349, "Control Mode"=w350, "PhoenixMotorControlDevRef"=w348) -> ("error out"=w346:errorcluster, "PhoenixMotorControlDevRef"=w347:T6)  [unwired: 6 in]
    }
    frame "New Testing Output" {
      w356 = T12 0 items=["PercentOutput"=0, "Position"=1, "Velocity"=2, "Current"=3, "Follower"=5, "MotionProfile"=6, "MotionMagic"=7, "MotionProfileArc"=10, "Disabled"=15] ("Control Mode")
      n114 = call <vilib>:"CTRE_Phoenix_MotorControl_Set.vi"("error in (no error)"=w353, "Output"=w354, "Control Mode"=w356, "PhoenixMotorControlDevRef"=w355) -> ("error out"=w351:errorcluster, "PhoenixMotorControlDevRef"=w352:T6)  [unwired: 6 in]
    }
  }
  n115 = case shown="\"New Normal Output\"" w34 {
    tunnel: w32 -> [_ w364 _]
    tunnel: w29 -> [w358 w362 w369]
    tunnel: w27 -> [_ w363 w368]
    tunnel: w30 -> [w357 w359 w367]
    tunnel: [w358 w361 w366] -> w28
    tunnel: [w357 w360 w365] -> _
    frame "No Changed Output", Default {
    }
    frame "New Normal Output" {
      n116 = call <vilib>:"CTRE_Phoenix_MotorControl_Set.vi"("error in (no error)"=w359, "Output"=w363, "Control Mode"=w364, "PhoenixMotorControlDevRef"=w362) -> ("error out"=w360:errorcluster, "PhoenixMotorControlDevRef"=w361:T6)  [unwired: 6 in]
    }
    frame "New Testing Output" {
      w370 = T12 0 items=["PercentOutput"=0, "Position"=1, "Velocity"=2, "Current"=3, "Follower"=5, "MotionProfile"=6, "MotionMagic"=7, "MotionProfileArc"=10, "Disabled"=15] ("Control Mode")
      n117 = call <vilib>:"CTRE_Phoenix_MotorControl_Set.vi"("error in (no error)"=w367, "Output"=w368, "Control Mode"=w370, "PhoenixMotorControlDevRef"=w369) -> ("error out"=w365:errorcluster, "PhoenixMotorControlDevRef"=w366:T6)  [unwired: 6 in]
    }
  }
  n118 = case shown="\"Module 3\"" "Plotting" {
    tunnel: w36 -> [_ w374 _ _ _]
    tunnel: [0.0 ("Interlock Output") w374 w376 w378 w380] -> w95
    tunnel: w35 -> [w371 w373 _ _ _]
    tunnel: [w371 w373 w375 w377 w379] -> w94
    tunnel: w27 -> [_ _ w376 _ _]
    tunnel: w28 -> [_ _ w375 _ _]
    tunnel: w20 -> [_ _ _ w378 _]
    tunnel: w19 -> [_ _ _ w377 _]
    tunnel: w12 -> [_ _ _ _ w380]
    tunnel: w11 -> [_ _ _ _ w379]
    frame "No Plot", Default {
    }
    frame "Module 0" {
    }
    frame "Module 1" {
    }
    frame "Module 2" {
    }
    frame "Module 3" {
    }
  }
  n119 = case shown="\"Module 0\"..\"Module 3\"" "Plotting" {
    tunnel: w95 -> [_ w391]
    tunnel: w94 -> [_ w392]
    frame "No Plot", Default {
    }
    frame "Module 0".."Module 3" {
      n120 = call-poly <vilib>:"CTRE_Phoenix_MotorController_Get_TalonFX.vi"("PhoenixMotorControlDevRef"=w392) -> ("Position (Raw Sensor Units)"=w396:i32, "Velocity (Raw Sensor Units per 100 ms)"=w395:i32)  [unwired: 11 in, 2 out]
      n121 = To Double Precision Float(number=w395) -> (double precision float=w394:dbl)
      n122 = To Double Precision Float(number=w396) -> (double precision float=w397:dbl)
      n123 = global read "robotconstants.vi" "Azimuth_Gear_Ratio"() -> (w381:dbl)
      n124 = expression code="360*x/(2048)" "counts to degrees"(w391) -> (w383:dbl)
      n125 = expression code="360*x/(2048)" "counts to degrees"(w397) -> (w387:dbl)
      n126 = expression code="(x*10*360)/(2048)" "convert from ticks/100ms to deg/s"(w394) -> (w385:dbl)
      n127 = Divide(x=w387, y=w381) -> (x/y=w386:dbl)
      n128 = Divide(x=w385, y=w381) -> (x/y=w384:dbl)
      n129 = Divide(x=w383, y=w381) -> (x/y=w382:dbl)
      n130 = Subtract(x=w386, y=w382) -> (x-y=w389:dbl)
      n131 = Bundle(w386, w382) -> (→"Azimuth Position":cluster{dbl, dbl})  [unwired: 1 in]
      n132 = Bundle(w384) -> (→"Azimuth Velocity":cluster{dbl})  [unwired: 1 in]
      n133 = Absolute Value(x=w389) -> (abs(x)=→"Azimuth Error (deg)":dbl)
    }
  }
